vi "Read Design Request.vi"(8 "error in":errorcluster, 11 "Master Method version":i32) -> (0 "error out":errorcluster, 1 "Number of Pending Requests":i32, 2 "Request Pending":bool, 3 "DesignRequest":T1, 4 "Method exists":bool, 6 "Successful Checkout":bool)   [LabVIEW 2011, in "Design Server.lvlib"]
uses:
  Design Server.lvlib
  Folders.ctl
  Variable cluster.ctl
  Design Request.ctl
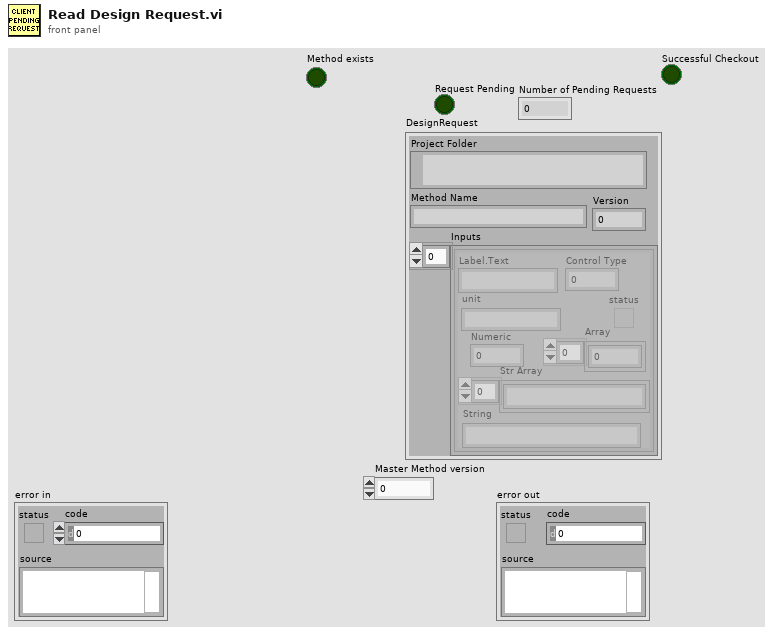
[diagram p1: front panel]
types:
  T1 = typedef "Design Server.lvlib/Design Request.ctl" = cluster{"Project Folder":path, "Method Name":string, "Inputs":T2, "Version":i32}
  T2 = typedef "Design Server.lvlib/Variable cluster.ctl" = cluster{"Label.Text":string, "Control Type":u32, "Numeric":dbl, "Array":dbl[], "status":bool, "Str Array":string[], "String":string, "unit":string}[]
  T3 = typedef "Design Server.lvlib/Folders.ctl" = enum16{"MathcadMethods", "RequestedDesigns", "CompletedDesigns", "MathcadCode", "CollabnetSVN.exe"}
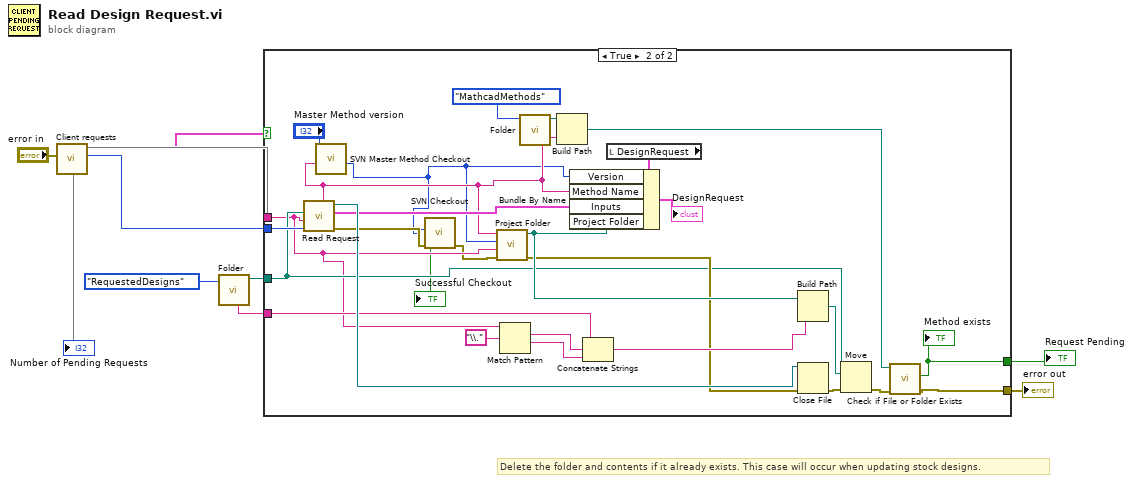
[diagram p0: block diagram]
diagram:
  # "Delete the folder and contents if it already exists. This case will occur when updating stock designs."
  n1 = call "Client requests.vi"(10:"error in") -> ("Number of Pending Requests"=w4:i32, "DesignRequest"=w3:T1, 5:w5, 7:→"Number of Pending Requests")  [unwired: 4 in, 3 out]
  n2 = call "Folder.vi"("Folders"=Folders."RequestedDesigns") -> ("FolderPath"=w7:path, "Folder name"=w6:string)  [unwired: 8 in, 1 out]
  n3 = case shown="True" w3 {
    selector: w3 -> [w11 _]
    tunnel: w5 -> [_ w19]
    tunnel: w4 -> [w12 w31]
    tunnel: [w12 w25] -> w10
    tunnel: [w11 w24] -> w9
    tunnel: w6 -> [_ w23]
    tunnel: w7 -> [_ w20]
    frame False {
    }
    frame True {
      n4 = call "Read Request.vi"("error in (no error)"=w31, "Request File Name"=w19, 10:w20) -> ("error out"=w18:errorcluster, "User and project info"=w32:T2, "Byte Stream File out"=w39:refnum<file>, "Method Name"=w15:string)  [unwired: 4 in, 1 out]
      n5 = call "SVN Master Method Checkout.vi"("Method Name"=w15, "Master Method version"="Master Method version") -> ("Method Version"=w13:i32)  [unwired: 5 in, 4 out]
      n6 = call "SVN Checkout.vi"("error in (no error)"=w18, "ADT version"=w13) -> ("error out"=w17:errorcluster, "Successful Checkout"=→"Successful Checkout":bool)  [unwired: 6 in, 2 out]
      n7 = call "Project Folder.vi"("error in (no error)"=w17, "Request File Name"=w19, "Revision"=w13, "Method"=w15) -> ("error out"=w21:errorcluster, "Completed Design path"=w22:path)  [unwired: 6 in]
      n8 = Match Pattern(string=w19, regular expression="\\.") -> (match substring=w36:string, after substring=w37:string)  [unwired: 1 in, 2 out]
      n9 = call "Folder.vi"("Folders"=Folders."MathcadMethods") -> ("FolderPath"=w30:path)  [unwired: 8 in, 2 out]
      n10 = Build Path(base path=w30, name or relative path=w15) -> (appended path=w27:path)
      n11 = Concatenate Strings(w23, w36, w37) -> (w35:string)
      n12 = local read "DesignRequest"() -> (w33:T1)
      n13 = Bundle By Name(cluster=w33, "Version"=w13, "Method Name"=w15, "Inputs"=w32, "Project Folder"=w22) -> (→"DesignRequest":T1)
      n14 = Build Path(base path=w22, name or relative path=w35) -> (appended path=w34:path)
      n15 = Close File(refnum=w39, error in=w21) -> (error out=w40:errorcluster)  [unwired: 1 out]
      n16 = Move(source path=w20, error in=w40, 10:w34) -> (error out=w26:errorcluster)  [unwired: 2 in, 2 out]
      n17 = call <vilib>:"Check if File or Folder Exists.vi"("error in (no error)"=w26, "path"=w27) -> ("error out"=w25:errorcluster, "file or folder exists?"=w24:bool)  [unwired: 7 in, 1 out]
      "Method exists" <- w24
    }
  }
  "Request Pending" <- w9
  "error out" <- w10
